vi "Test 2 Get STart.vi"(8 "error in (no error)":errorcluster, 11 "Test Case In":refnum<class "Day X Test.lvclass">) -> (0 "error out":errorcluster, 3 "Test Case Out":refnum<class "Day X Test.lvclass">)   [LabVIEW 2020, in "Day X Test.lvclass"]
uses:
  Day X Test.lvclass
  C:/Program Files (x86)/National Instruments/LabVIEW 2020/vi.lib/Astemes/LUnit/Test Case.lvclass
  <vilib>/Astemes/LUnit/Test Case.lvclass/Test Case.ctl
  4993e8ee-a06a-463a-9684-69129f64d5ce.vi
  b710daaf-7c26-4ab2-82e8-49672fcae945.vi
  <vilib>/Astemes/LUnit/Append Pass Result.vi
  <vilib>/Astemes/LUnit/Append Fail Result.vi
  <vilib>/Astemes/LUnit/Describe Comparison.vi
  <vilib>/Astemes/LUnit/Compare Variants.vi
  <vilib>/Astemes/LUnit/Variant to string.vi
  <vilib>/Utility/Data Type/Get Type Information.vi
  <vilib>/Utility/LVClass/Get LV Class Name.vi
  Map/Maze.lvclass
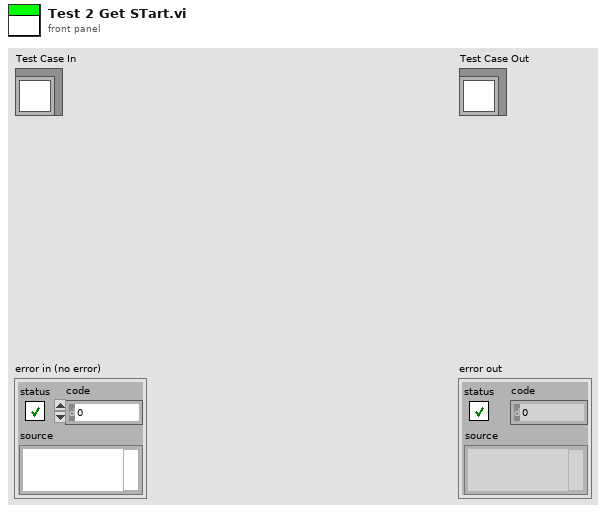
[diagram p1: front panel]
types:
  T1 = typedef "Maze.lvclass/Position.ctl" = cluster{"Row":u64, "Col":u64, "Next Move":enum16{"North", "East", "South", "West", "Halt"}}
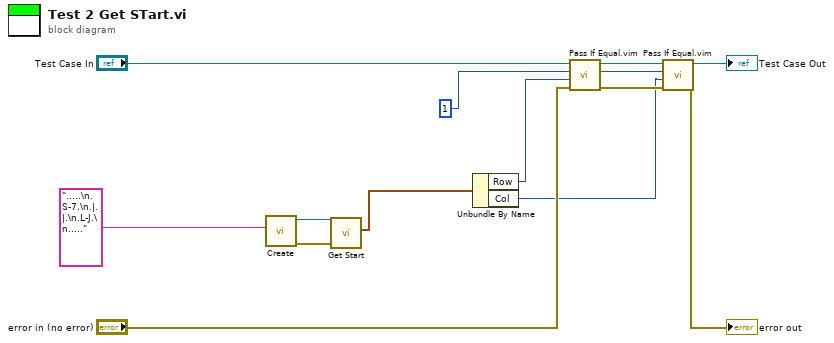
[diagram p0: block diagram]
diagram:
  w4 = u64 1 ("Row")
  n1 = call "Create.vi"("Input"=".....\n.S-7.\n.|.|.\n.L-J.\n.....") -> ("error out"=w9:errorcluster, "Map"=w10:refnum<class "Maze.lvclass">)  [unwired: 9 in]
  n2 = call "Get Start.vi"("error in (no error)"=w9, "Map in"=w10) -> ("Start Vectors"=w3:T1)  [unwired: 7 in, 2 out]
  n3 = Unbundle By Name(w3) -> ("Row"=w2:u64, "Col"=w1:u64)
  n4 = call "Pass If Equal.vim"("error in (no error)"="error in (no error)", "Actual"=w2, "Expected"=w4, "LUnit Test Case In"="Test Case In") -> ("error out"=w8:errorcluster, "LUnit Test Case Out"=w6:refnum<class "Day X Test.lvclass">)  [unwired: 6 in]
  n5 = call "Pass If Equal.vim"("error in (no error)"=w8, "Actual"=w1, "Expected"=w4, "LUnit Test Case In"=w6) -> ("error out"=→"error out":errorcluster, "LUnit Test Case Out"=→"Test Case Out":refnum<class "Day X Test.lvclass">)  [unwired: 6 in]
